vi "Element Type.vi"(11 "NumericIndicator in":refnum<class "NumericIndicator.lvclass">) -> (2 "Element Type":string)   [LabVIEW 2020, in "VolatusGUI.lvlib" / "NumericIndicator.lvclass"]
uses:
  NumericIndicator.lvclass
  NumericIndicator.lvclass/NumericIndicator.ctl
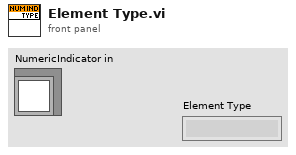
[diagram p1: front panel]
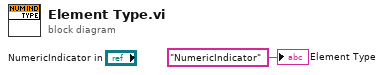
[diagram p0: block diagram]
diagram:
  "Element Type" <- "NumericIndicator" ("Indicator Type")
